vi "ACIR Channel UI.vi"() -> ()   [LabVIEW 2025, in "ACIR.lvlib" / "ACIR Channel.lvclass"]
doc: "Copyright 2017 National Instruments Corporation\n\nLicensed under the Apache License, Version 2.0 (the \"License\"); you may not use this file except in compliance with the License. You may obtain a copy of the License at http://www.apache.org/licenses/LICENSE-2.0\nUnless required by applicable law or agreed to in writing, software distributed under the License is distributed on an \"AS IS\" BASIS, WITHOUT WARRANTIES OR CONDITIONS OF ANY KIND, either express or implied. See the License for the specific language governing permissions and limitations under the License."
uses:
  ACIR Channel.lvclass
  Users/Public/Documents/Sandia National Labs/TSS Plugin/CEF.lvlibp/Node/NodeRef.ctl
  Users/Public/Documents/Sandia National Labs/TSS Plugin/CEF.lvlibp/Node/CEF_Node.lvclass
  Users/Public/Documents/Sandia National Labs/TSS Plugin/CEF.lvlibp/Node/mainQref.ctl
  Users/Public/Documents/Sandia National Labs/TSS Plugin/CEF.lvlibp/Node/UserEventRef.ctl
  Users/Public/Documents/Sandia National Labs/TSS Plugin/Abstract Engine.lvlibp/Plugin/Abstract/Channel configuration/Default Channel.ctl
  ACIR Channel.lvclass/ACIR Channel.ctl
  <vilib>/Utility/error.llb/Trim Whitespace One-Sided.vi
  Users/Public/Documents/Sandia National Labs/TSS Plugin/Abstract Engine.lvlibp/Plugin/Abstract/Channel configuration/Read Channel Setting.vi
  Users/Public/Documents/Sandia National Labs/TSS Plugin/Abstract Engine.lvlibp/Plugin/Abstract/Channel configuration/Write Channel Setting.vi
  Users/Public/Documents/Sandia National Labs/TSS Plugin/Abstract Engine.lvlibp/Plugin/Abstract/Channel configuration/Channel configuration.lvclass
panel:
  in  "ACIR Channel":T1={"Address"="None", "SW Alias"="None", "Enabled"=TRUE, "Type"="None", "Description"="* Type = Channel Class"}
  in  "user event":T2
  in  "main queue":T3
  in  "node ref":T4
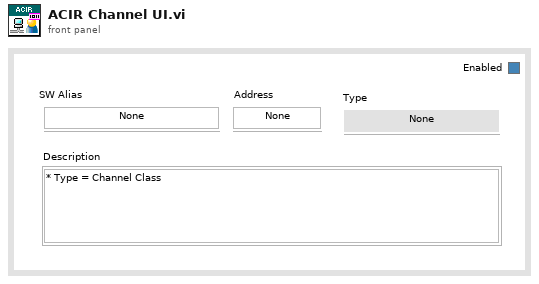
[diagram p1: front panel]
types:
  T1 = typedef "Abstract Engine.lvlibp/Channel configuration.lvclass/Default Channel.ctl" = cluster{"Address":string, "SW Alias":string, "Enabled":bool, "Type":string, "Description":string}
  T2 = typedef "CEF.lvlibp/CEF_Node.lvclass/UserEventRef.ctl" = refnum<user-event>
  T3 = typedef "CEF.lvlibp/CEF_Node.lvclass/mainQref.ctl" = refnum<queue>
  T4 = typedef "CEF.lvlibp/CEF_Node.lvclass/NodeRef.ctl" = refnum<data-value>
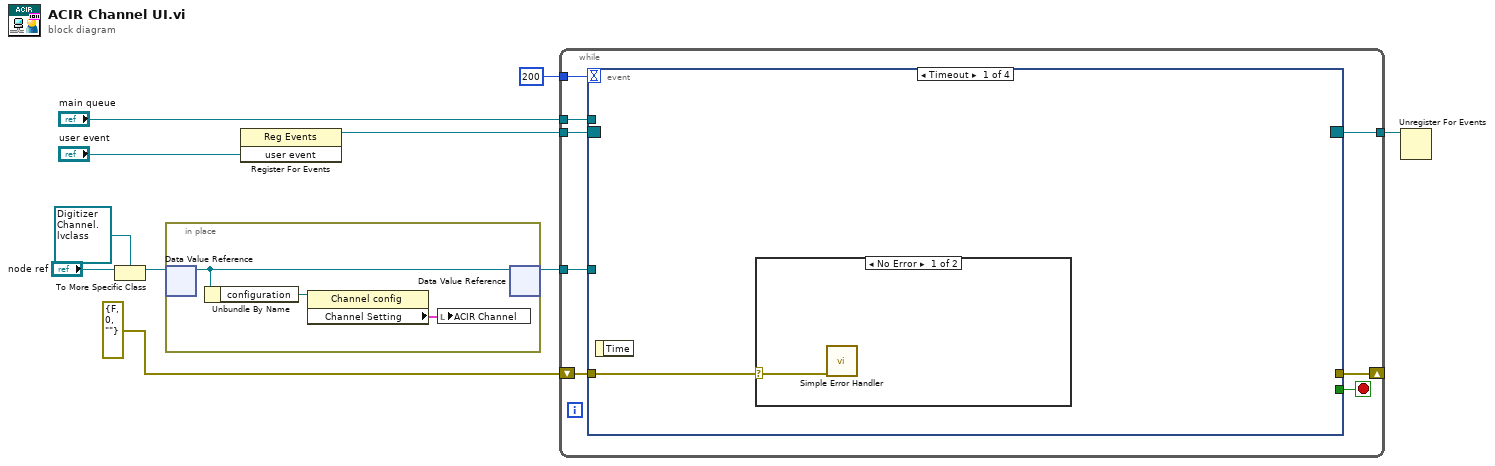
[diagram p0: block diagram]
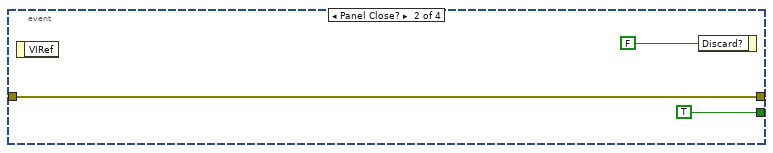
[diagram p3: hidden frame]
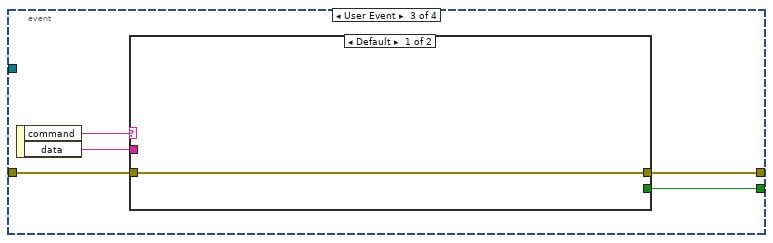
[diagram p4: hidden frame]
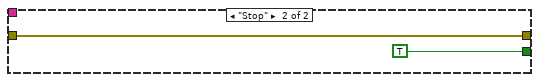
[diagram p5: hidden frame]
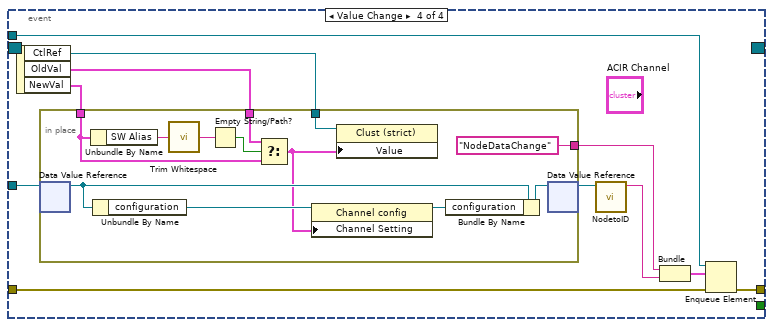
[diagram p6: hidden frame]
diagram:
  n1 = To More Specific Class(target class=refnum<data-value> refnum ("data value reference"), reference="node ref") -> (specific class reference=w5:refnum<data-value>)  [unwired: 1 in, 1 out]
  n2 = in-place {
    # "Initialize the front panel controls when loaded"
    n3 = in-place-dvr #1(w5) -> (w13:refnum<class "ACIR Channel.lvclass">)  [unwired: 1 out]
    n4 = Unbundle By Name(w13) -> ("configuration"=w12:refnum<class "Channel configuration.lvclass">)
    n5 = property class="Channel config"(reference=w12) -> ("Channel Setting"=w11:T1)  [unwired: 1 in, 2 out]
    n6 = local write "ACIR Channel"(w11) -> ()
    n7 = in-place-dvr #1(w13) -> (w4:refnum<data-value>)  [unwired: 1 out]
  }
  n8 = register-events("user event") -> (reference out=w9:refnum<event-registration>)  [unwired: 2 in, 1 out]
  n9 = while {
    tunnel: w4 -> [w21]
    tunnel: w9 -> [w20]
    tunnel: [w19] -> w8
    tunnel: "main queue" -> [w15]
    shift-right: [w16] -> _
    shift-left: errorcluster {"status"=FALSE, "code"=0, "source"=""} ("error out") -> [w17]
    tunnel: 200 -> [w14]
    stop <- w18 stop-if-true
    n10 = event shown="[0] Timeout" {
      selector: w20 -> [_ _ _ _]
      dyn-events: [_ _ _ _] -> w19
      timeout: w14 -> [_ _ _ _]
      tunnel: w21 -> [_ _ _ w44]
      tunnel: [_ TRUE w31 _] -> w18
      tunnel: [_ w24 w27 w45] -> w16
      tunnel: w17 -> [w22 w24 w29 w38]
      tunnel: w15 -> [_ _ _ w39]
      event Timeout {
        n11 = event-data() -> ()  [unwired: 1 in, 1 out]
        n12 = case shown="No Error" w22 {
          selector: w22 -> [w23 _]
          frame No Error {
            n13 = call <vilib>:"Simple Error Handler.vi"("error in (no error)"=w23) -> ()  [unwired: 4 in, 5 out]
          }
          frame Error {
          }
        }
      }
      event Panel Close? {
        n14 = event-data() -> ()  [unwired: 1 in, 1 out]
        n15 = event-data("Discard?"=FALSE) -> ()  [unwired: 1 in, 1 out]
      }
      event User Event {
        n16 = event-data() -> ("command"=w28:string, "data"=w30:string)  [unwired: 1 in]
        n17 = case shown="Default" w28 {
          tunnel: [_ TRUE] -> w31
          tunnel: w30 -> [_ _]
          tunnel: w29 -> [w32 w33]
          tunnel: [w32 w33] -> w27
          frame Default {
          }
          frame "Stop" {
          }
        }
      }
      event Value Change {
        n18 = event-data() -> ("CtlRef"=w40:refnum<vi>, "OldVal"=w41:T1, "NewVal"=w42:T1)  [unwired: 1 in]
        n19 = in-place {
          in-place-border: w42 -> [w51]
          in-place-border: w41 -> [w54]
          in-place-border: w40 -> [w53]
          in-place-border: ["NodeDataChange" ("Message Name")] -> w36
          n20 = in-place-dvr #2(w44) -> (w57:refnum<class "ACIR Channel.lvclass">)  [unwired: 1 out]
          n21 = Unbundle By Name(w51) -> ("SW Alias"=w52:string)
          n22 = Unbundle By Name(w57) -> ("configuration"=w48:refnum<class "Channel configuration.lvclass">)
          n23 = call <vilib>:"Trim Whitespace.vi"("string"=w52) -> ("trimmed string"=w49:string)  [unwired: 1 in]
          n24 = Empty String/Path?(string/path=w49) -> (empty?=w50:bool)
          n25 = Select(t=w54, s=w50, f=w51) -> (s? t:f=w46:T1)
          n26 = property class="Channel config"(reference=w48, "Channel Setting"=w46) -> (reference out=w55:refnum<class "Channel configuration.lvclass">)  [unwired: 1 in, 1 out]
          n27 = property class="Clust (strict)"(reference=w53, "Value"=w46) -> ()  [unwired: 1 in, 2 out]
          n28 = Bundle By Name(cluster=w57, "configuration"=w55) -> (w56:refnum<class "ACIR Channel.lvclass">)
          n29 = in-place-dvr #2(w56) -> (w43:refnum<data-value>)  [unwired: 1 out]
        }
        n30 = call "NodetoID.vi"("node ref"=w43) -> ("ID"=w37:string)  [unwired: 9 in, 1 out]
        n31 = Bundle("Message Name"=w36, "ID"=w37) -> (w35:cluster{"Message Name":string, "ID":string})  [unwired: 1 in]
        n32 = Enqueue Element(queue=w39, element=w35, error in (no error)=w38) -> (error out=w45:errorcluster)  [unwired: 1 in, 2 out]
      }
    }
  }
  n33 = Unregister For Events(event registration refnum=w8) -> ()  [unwired: 1 in, 1 out]
